vi "last 10 values as an action engine.vi"(7 "read write":enum16{"Read", "Write"}(ring), 11 "last 10 values Write":T1) -> (3 "last 10 values read":T1)   [LabVIEW 2010]
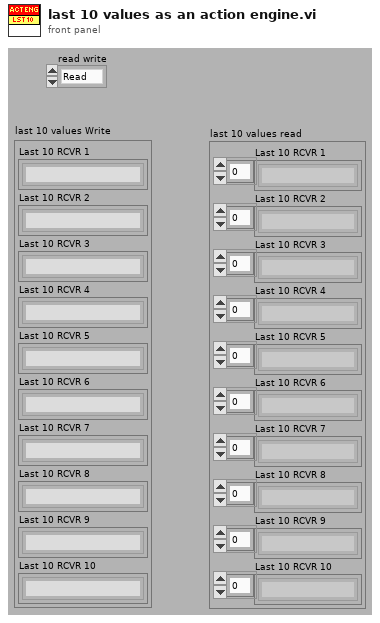
[diagram p1: front panel]
types:
  T1 = cluster{"Last 10 RCVR 1":string[], "Last 10 RCVR 2":string[], "Last 10 RCVR 3":string[], "Last 10 RCVR 4":string[], "Last 10 RCVR 5":string[], "Last 10 RCVR 6":string[], "Last 10 RCVR 7":string[], "Last 10 RCVR 8":string[], "Last 10 RCVR 9":string[], "Last 10 RCVR 10":string[]}
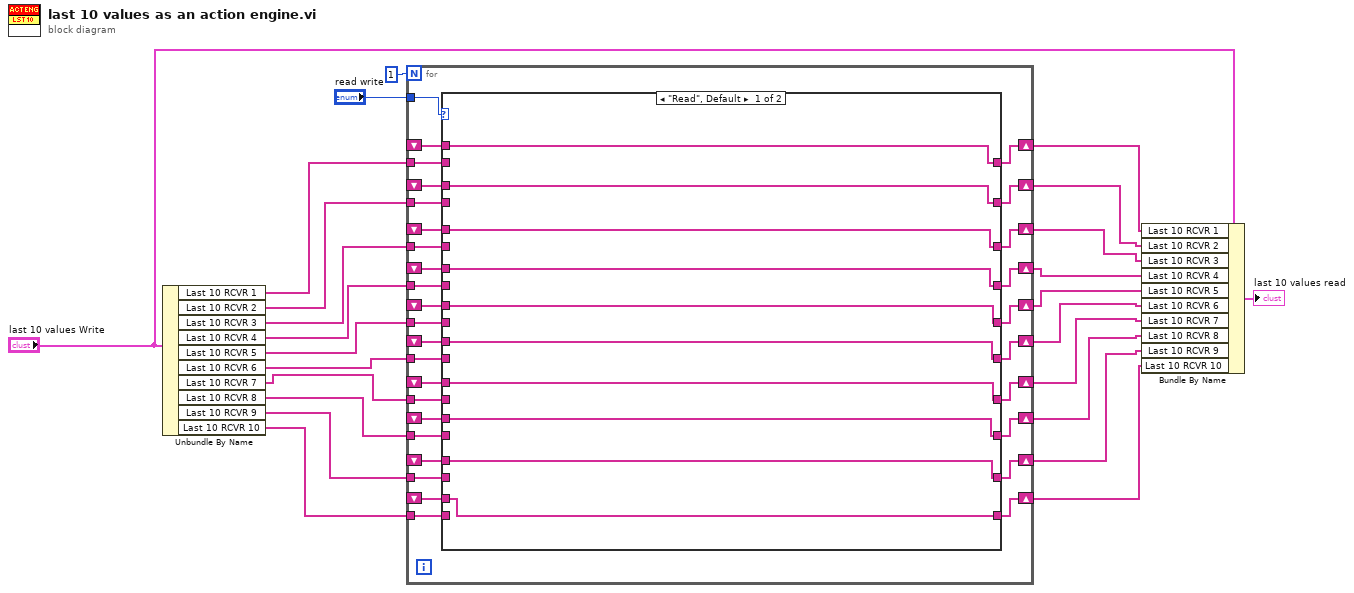
[diagram p0: block diagram]
diagram:
  n1 = Unbundle By Name("last 10 values Write") -> ("Last 10 RCVR 1"=w22:string[], "Last 10 RCVR 2"=w21:string[], "Last 10 RCVR 3"=w20:string[], "Last 10 RCVR 4"=w19:string[], "Last 10 RCVR 5"=w18:string[], "Last 10 RCVR 6"=w17:string[], "Last 10 RCVR 7"=w16:string[], "Last 10 RCVR 8"=w15:string[], "Last 10 RCVR 9"=w14:string[], "Last 10 RCVR 10"=w13:string[])
  n2 = for {
    N: 1 -> [_]
    tunnel: "read write" -> [w55]
    tunnel: w22 -> [w54]
    shift-right: [w53] -> w11
    shift-left: _ -> [w52]
    tunnel: w21 -> [w49]
    shift-right: [w50] -> w10
    shift-left: _ -> [w51]
    tunnel: w20 -> [w48]
    shift-right: [w47] -> w9
    shift-left: _ -> [w46]
    tunnel: w19 -> [w43]
    shift-right: [w44] -> w8
    shift-left: _ -> [w45]
    tunnel: w18 -> [w42]
    shift-right: [w41] -> w7
    shift-left: _ -> [w40]
    tunnel: w17 -> [w37]
    shift-right: [w38] -> w6
    shift-left: _ -> [w39]
    tunnel: w16 -> [w36]
    shift-right: [w35] -> w5
    shift-left: _ -> [w34]
    tunnel: w15 -> [w31]
    shift-right: [w32] -> w4
    shift-left: _ -> [w33]
    tunnel: w14 -> [w30]
    shift-right: [w29] -> w3
    shift-left: _ -> [w28]
    tunnel: w13 -> [w25]
    shift-right: [w26] -> w2
    shift-left: _ -> [w27]
    n3 = case shown="\"Read\", Default" w55 {
      tunnel: w54 -> [_ w75]
      tunnel: [w65 w75] -> w53
      tunnel: w52 -> [w65 _]
      tunnel: w49 -> [_ w74]
      tunnel: [w64 w74] -> w50
      tunnel: w51 -> [w64 _]
      tunnel: w48 -> [_ w73]
      tunnel: [w63 w73] -> w47
      tunnel: w46 -> [w63 _]
      tunnel: w43 -> [_ w72]
      tunnel: [w62 w72] -> w44
      tunnel: w45 -> [w62 _]
      tunnel: w42 -> [_ w71]
      tunnel: [w61 w71] -> w41
      tunnel: w40 -> [w61 _]
      tunnel: w37 -> [_ w70]
      tunnel: [w60 w70] -> w38
      tunnel: w39 -> [w60 _]
      tunnel: w36 -> [_ w69]
      tunnel: [w59 w69] -> w35
      tunnel: w34 -> [w59 _]
      tunnel: w31 -> [_ w68]
      tunnel: [w58 w68] -> w32
      tunnel: w33 -> [w58 _]
      tunnel: w30 -> [_ w67]
      tunnel: [w57 w67] -> w29
      tunnel: w28 -> [w57 _]
      tunnel: w25 -> [_ w66]
      tunnel: [w56 w66] -> w26
      tunnel: w27 -> [w56 _]
      frame "Read", Default {
      }
      frame "Write" {
      }
    }
  }
  n4 = Bundle By Name(cluster="last 10 values Write", "Last 10 RCVR 1"=w11, "Last 10 RCVR 2"=w10, "Last 10 RCVR 3"=w9, "Last 10 RCVR 4"=w8, "Last 10 RCVR 5"=w7, "Last 10 RCVR 6"=w6, "Last 10 RCVR 7"=w5, "Last 10 RCVR 8"=w4, "Last 10 RCVR 9"=w3, "Last 10 RCVR 10"=w2) -> (→"last 10 values read":T1)
